vi "GetOperatingMode.vi"(0 "VISA resource name":refnum<visa-resource-name>, 11 "error in":errorcluster) -> (4 "VISA resource name out":refnum<visa-resource-name>, 6 "Operating mode string":string, 8 "Operating mode":u8, 10 "Operating mode binary":string, 15 "error out":errorcluster)   [LabVIEW 2023, in "Thermotron 8800.lvlib"]
doc: "MODE\nCommand name: Send operating mode of 8800\nCommand type: System status\nDescription: The query command asks the 8800 for its current operating mode.\nSyntax: MODE?\nThe 8800 will respond to this query command with a coded integer byte:\nBits 0 through 7\nBit 0 Program mode \nBit 1 Edit mode (controller in stop mode) \nBit 2 View program mode \nBit 3 Edit mode (controller in hold mode) \nBit 4 Manual mode \nBit 5 Delayed start mode \nBit 6 Unused \nBit 7 Calibration mode\nData type: Coded integer\nQuery example: Mode?\n8800 response: 0 (The 8800 is in program mode.)"
uses:
  Thermotron 8800.lvlib
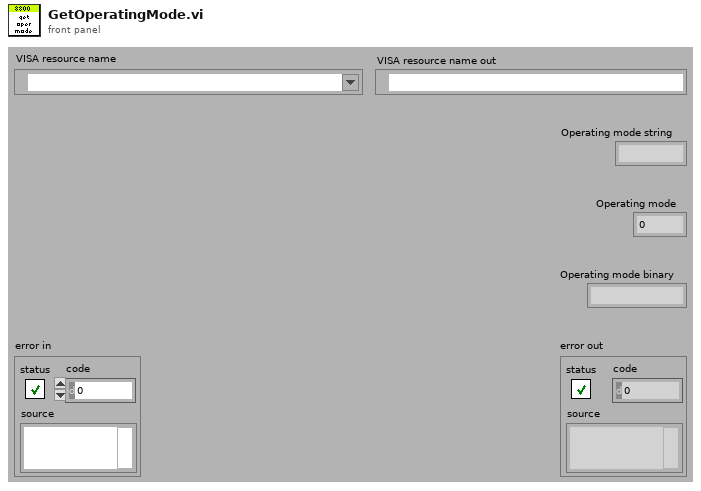
[diagram p1: front panel]
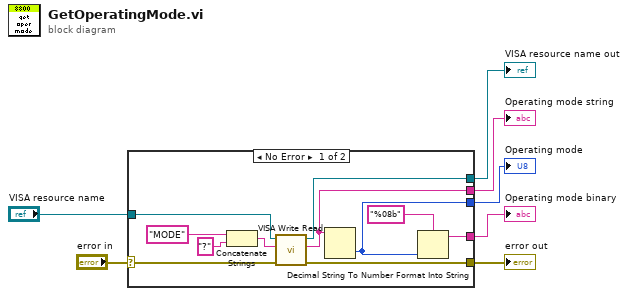
[diagram p0: block diagram]
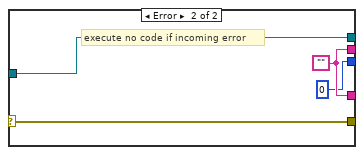
[diagram p2: hidden frame]
diagram:
  n1 = case shown="No Error" "error in" {
    selector: "error in" -> [w15 w21]
    tunnel: [w12 w21] -> w6
    tunnel: [w13 w22] -> w5
    tunnel: "VISA resource name" -> [w14 w22]
    tunnel: [w11 w20] -> w3
    tunnel: [w9 w20] -> w2
    tunnel: [w8 0] -> w1
    frame No Error {
      n2 = Concatenate Strings("MODE" ("8800 Command"), "?" ("8800 Command")) -> (w18:string)
      n3 = call "VISA Write Read.vi"("error in (no error)"=w15, "8800 Command"=w18, "VISA Refnum in"=w14) -> ("error out"=w12:errorcluster, "read buffer"=w11:string, "VISA Refnum out"=w13:refnum<visa-resource-name>)  [unwired: 6 in]
      n4 = Decimal String To Number(string=w11) -> (number=w8:i32)  [unwired: 2 in, 1 out]
      n5 = Format Into String(format string="%08b", w8) -> (resulting string=w9:string)  [unwired: 2 in, 1 out]
    }
    frame Error {
      w20 = ""
      # "execute no code if incoming error"
    }
  }
  "VISA resource name out" <- w5
  "error out" <- w6
  "Operating mode string" <- w3
  "Operating mode binary" <- w2
  "Operating mode" <- w1
